vi "Wiggle Actuators.vi"(10 "Trigger":dbl) -> (2 "MotorCommand":dbl)   [LabVIEW 2014]
panel:
  # "This Vi runs an oscillating motor setpoint\nthru actuator to move rudder and prop\nduring initialization state"
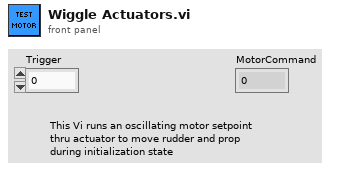
[diagram p1: front panel]
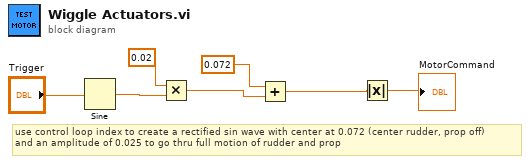
[diagram p0: block diagram]
diagram:
  # "use control loop index to create a rectified sin wave with center at 0.072 (center rudder, prop off)\nand an amplitude of 0.025 to go thru full motion of rudder and prop"
  n1 = Sine(x="Trigger") -> (sin(x)=w6:dbl)
  n2 = Multiply(x=0.02, y=w6) -> (x*y=w3:dbl)
  n3 = Add(x=0.072, y=w3) -> (x+y=w1:dbl)
  n4 = Absolute Value(x=w1) -> (abs(x)=→"MotorCommand":dbl)
